vi "Create Execution Unit.vi"(8 "error in":errorcluster, 10 "Item Ref":T1=18446744073709551615 format="%.0x", 11 "Execution Unit Factory Implementation in":refnum<class "Execution Unit Factory Implementation.lvclass">) -> (0 "error out":errorcluster, 2 "Execution Unit Information":T2 {"Outgoing Channels" format="%.0x"; "Incoming Channels" format="%.0x"}, 3 "Execution Unit Factory Implementation out":refnum<class "Execution Unit Factory Implementation.lvclass">)   [LabVIEW 2020, in "Communication Bus Template Interfaces.lvlib" / "Protocol Implementation.lvlib" / "Execution Unit Factory Implementation.lvclass"]
uses:
  Execution Unit Factory Implementation.lvclass
  Interfaces/Execution Unit/Execution Unit Information.ctl
  Interfaces/Execution Unit/Execution Unit/Execution Unit.lvclass
  <vilib>/NI VeriStand/Custom Device API/Custom Device Item Ref.ctl
  Execution Unit Implementation/Execution Unit Implementation.lvclass
  C:/Dev/GitHub/niveristand-communications-bus-template/Source/Interfaces/Execution Unit/Execution Unit/Execution Unit.lvclass
  <vilib>/NI VeriStand/Custom Device API/Custom Device API.lvlib
  Interfaces/Execution Unit/Execution Unit.lvlib
  C:/Dev/GitHub/niveristand-communications-bus-template/Source/Implementation/Execution Unit Implementation/Execution Unit Implementation.lvclass
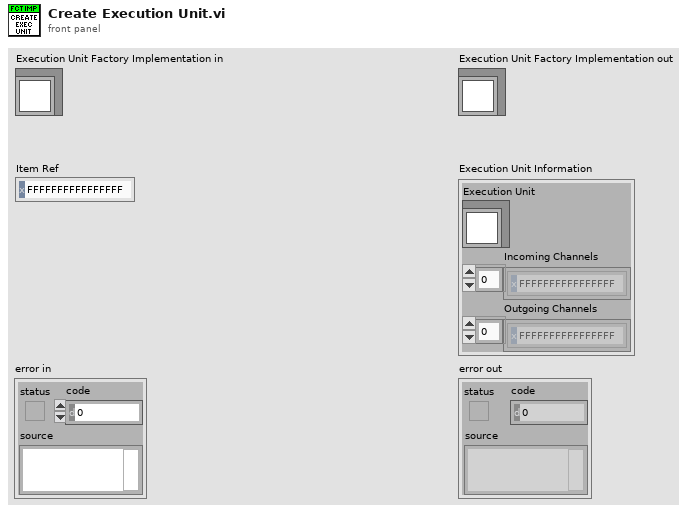
[diagram p1: front panel]
types:
  T1 = typedef "Custom Device API.lvlib/Custom Device Item Ref.ctl" = u64
  T2 = typedef "Communication Bus Template Interfaces.lvlib/Execution Unit.lvlib/Execution Unit Information.ctl" = cluster{"Execution Unit":refnum<class "Execution Unit.lvclass">, "Incoming Channels":T1[], "Outgoing Channels":T1[]}
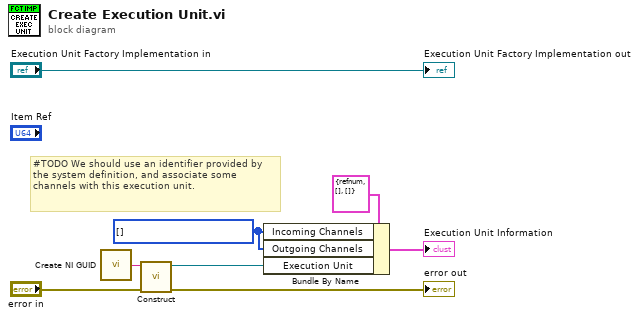
[diagram p0: block diagram]
diagram:
  w6 = T1[] [] ("Incoming Channels")
  # "#TODO We should use an identifier provided by the system definition, and associate some channels with this execution unit."
  n1 = call <vilib>:"Create NI GUID.vi"() -> ("NI GUID"=w1:string)
  n2 = call "Construct.vi"("error in (no error)"="error in", "id"=w1) -> ("error out"=→"error out":errorcluster, "Execution Unit Implementation"=w2:refnum<class "Execution Unit Implementation.lvclass">)  [unwired: 8 in]
  n3 = Bundle By Name(cluster=T2 {"Execution Unit"=refnum, "Incoming Channels"=[], "Outgoing Channels"=[]} ("Execution Unit Information"), "Incoming Channels"=w6, "Outgoing Channels"=w6, "Execution Unit"=w2) -> (→"Execution Unit Information":T2)
  "Execution Unit Factory Implementation out" <- "Execution Unit Factory Implementation in"
